vi "Little-Endian Bytes To Words I64.vi"(1 "bytes in":u8[](array[numeric]) format="%02x") -> (0 "words out":i64[](array[numeric]))   [LabVIEW 2020, in "NI_Bit Manipulation.lvlib"]
uses:
  <vilib>/Bit Manipulation/NI_Bit Manipulation.lvlib
  068ac748-d2cd-4c9a-8044-fc563640b5b0.vi
  068ac748-d2cd-4c9a-8044-fc563640b5b0.vi/4b48189a-3f55-41bb-b295-66cadd48166d.vi
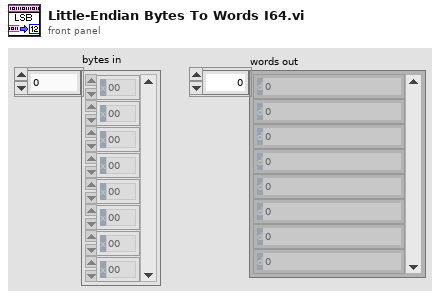
[diagram p1: front panel]
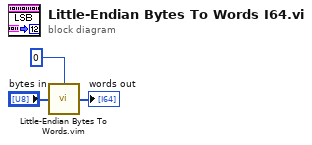
[diagram p0: block diagram]
diagram:
  n1 = call "Little-Endian Bytes To Words.vim"("bytes in"="bytes in", "word type"=i64 0) -> ("words out"=→"words out":i64[])
